vi "TS - Read controller status.vi"(2 "error in":errorcluster, 3 "Address / Port":i16=1 min=1 max=31 step=1) -> (0 "error out":errorcluster, 1 "Read the controller status\nbyte in ASCII":string)   [LabVIEW 2014]
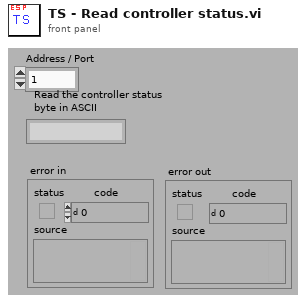
[diagram p1: front panel]
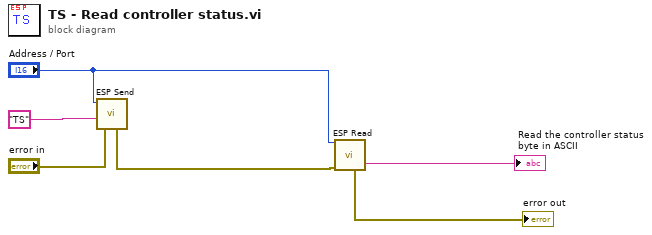
[diagram p0: block diagram]
diagram:
  n1 = call "ESP Send.vi"("Address / Port"="Address / Port", "Command String"="TS" ("Substring"), "error in"="error in") -> ("error out"=w4:errorcluster)  [unwired: 5 in]
  n2 = call "ESP Read.vi"("Address / Port"="Address / Port", "error in"=w4) -> ("error out"=→"error out":errorcluster, "Response String"=→"Read the controller status\nbyte in ASCII":string)  [unwired: 5 in]
